vi "Read Update Period.vi"(8 "error in (no error)":errorcluster, 11 "Content in":refnum<class "Content.lvclass">) -> (0 "error out":errorcluster, 2 "Update Period":dbl, 3 "Content out":refnum<class "Content.lvclass">)   [LabVIEW 2026, in "LED Matrix.lvlib" / "Content.lvclass"]
uses:
  Content.lvclass
  Content.lvclass/Content.ctl
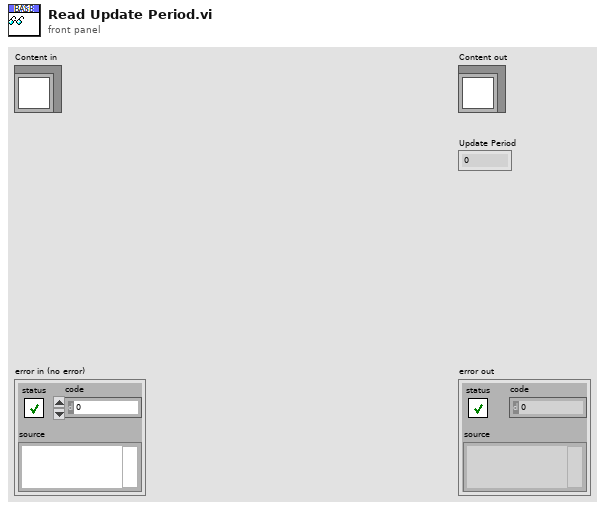
[diagram p1: front panel]
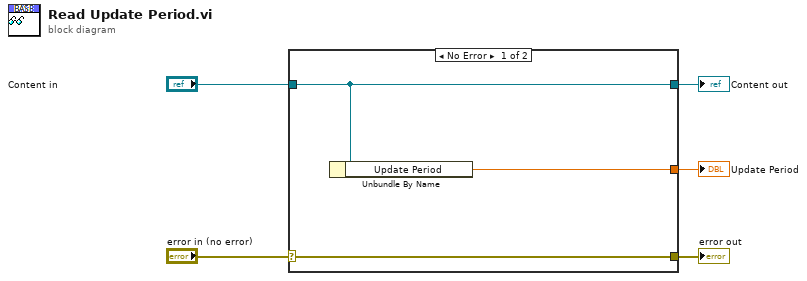
[diagram p0: block diagram]
diagram:
  n1 = case shown="No Error" "error in (no error)" {
    selector: "error in (no error)" -> [w8 w9]
    tunnel: [w8 w9] -> w4
    tunnel: [w7 w10] -> w2
    tunnel: "Content in" -> [w7 w10]
    tunnel: [w6 _] -> w1
    frame No Error {
      n2 = Unbundle By Name(w7) -> ("Update Period"=w6:dbl)
    }
    frame Error {
    }
  }
  "error out" <- w4
  "Content out" <- w2
  "Update Period" <- w1
